vi "dev_generate-fake.vi"() -> (3 "Array":dbl[](array[numeric]))   [LabVIEW 2024]
uses:
  <vilib>/Analysis/NI_AALBase.lvlib
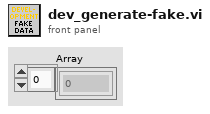
[diagram p1: front panel]
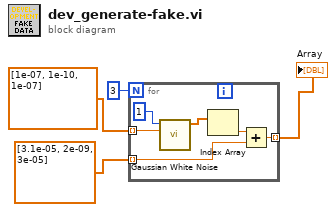
[diagram p0: block diagram]
diagram:
  n1 = for {
    N: 3 -> [_]
    tunnel: dbl[] [3.1e-05, 2e-09, 3e-05] ("y") -> [w10] mode=indexing
    tunnel: [w9] -> w2 mode=indexing
    tunnel: dbl[] [1e-07, 1e-10, 1e-07] ("standard deviation") -> [w7] mode=indexing
    n2 = call <vilib>:"Gaussian White Noise.vi"("standard deviation"=w7, "samples"=1) -> ("Gaussian noise pattern"=w6:dbl[])  [unwired: 8 in, 1 out]
    n3 = Index Array(array=w6) -> (element=w5:dbl)  [unwired: 1 in]
    n4 = Add(x=w5, y=w10) -> (x+y=w9:dbl)
  }
  "Array" <- w2
